vi "VI Test.vi"(6 "Aktion":T1, 8 "error in (no error)":errorcluster caption="Fehler (Eingang, kein Fehler)") -> (0 "error out":errorcluster caption="Fehler (Ausgang)", 1 "Status Test":string, 2 "Fertig":bool, 4 "Aktion":T1, 5 "Test":dbl=30.0, 7 "Warten":dbl)   [LabVIEW 2020, in "EPA 1065.lvlib" / "Interference verificaton 1065-366.lvlib"]
uses:
  Interference verificaton 1065-366.lvlib
  Aktion Test.ctl
  Sprachverwaltung/FGV Aktion Tabelle zerlegen.ctl
  Aktion FGV Interference.ctl
  Aktion Index uebersetzten.ctl
  Seiten/CalGas Aufschaltung/FGV CalGas Aktionen.ctl
  Funktionstasten/Zustaende.ctl
  Funktionstasten/Funktionstasten-Aktion.ctl
  Seiten/CalGas Aufschaltung/Auswahl Aufschaltpunkt.ctl
  PNS/Aktionen FGV Grenzwerte.ctl
  Sprachverwaltung/Sprachverwaltung.lvlib
  Funktionstasten/Funktionstasten.lvlib
  Seiten/CalGas Aufschaltung/CalGas Aufschaltung.lvlib
  PNS/PNS.lvlib
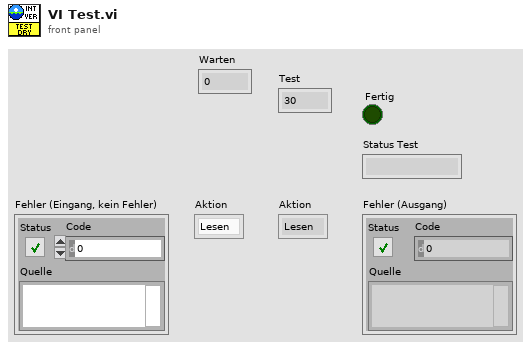
[diagram p1: front panel]
types:
  T1 = typedef "EPA 1065.lvlib/Interference verificaton 1065-366.lvlib/Aktion Test.ctl" = enum16{"Lesen", "ini", "ini - Konz", "Konzentration erreicht", "ini-warten", "ini-Warten-Stabil", "Warten-Stabil", "ini-warten-aufzeichnen", "Warten-Aufzeichnen", "aufzeichnen", "ini-wet", "ini - konz - wet", "Konzentration erreicht - wet", "ini - warten - wet", "warten - wet", "warten - aufzeichnen - wet", "Auswerten", "aufzeichnen - wet"}
  T2 = typedef "CalGas Aufschaltung.lvlib/FGV CalGas Aktionen.ctl" = enum16{"lesen", "Analysator Auswahl", "Def.CalGas", "Aufschaltung CalGas", "laden", "speichern", "KAL extrahieren"}
  T3 = typedef "EPA 1065.lvlib/Interference verificaton 1065-366.lvlib/Aktion Index uebersetzten.ctl" = enum16{"lesen", "schreiben", "auswerten"}
  T4 = typedef "EPA 1065.lvlib/Interference verificaton 1065-366.lvlib/Aktion FGV Interference.ctl" = enum16{"Lesen", "TestKonfig", "TestSetting", "Einheiten", "Ergebnis", "Laden", "Tabelle", "Speichern", "löschen"}
  T5 = typedef "Sprachverwaltung.lvlib/FGV Aktion Tabelle zerlegen.ctl" = enum16{"laden", "vereinzeln", "speichern"}
  T6 = typedef "Funktionstasten.lvlib/Funktionstasten-Aktion.ctl" = enum16{"Initialisieren", "Zustand setzen", "Taste gedrückt", "Fehler speichern", "Lesen", "Manuell", "Remote", "Bitparallel", "Samplepoint", "Zeit Prüfen", "reset Umschalten"}
  T7 = typedef "Funktionstasten.lvlib/Zustaende.ctl" = enum16{"Standby", "Pause", "Eco", "Messen", "Kalibrieren", "Spülen Filter", "Spülen Leitung", "Umgebungsluft", "0-Gas", "Cal-Gas", "CG zu PNS", "-------------", "Init 1", "Init 2", "Init 3", "Init 4", "Messen vorbereiten", "Messen durchführen", "Exit"}
  T8 = typedef "CalGas Aufschaltung.lvlib/Auswahl Aufschaltpunkt.ctl" = enum16{"über Filterblock", "Analysator direkt", "über PNS", "Entnahme", "Gasdivider"}
  T9 = typedef "PNS.lvlib/Aktionen FGV Grenzwerte.ctl" = enum16{"lesen", "Grenzw. schreiben", "Anweisungscode", "IP-Adresse", "laden", "speichern", "Anweisungscode vorgeben"}
  T10 = typedef "CalGas Aufschaltung.lvlib/Aufschaltung CalGas.ctl" = cluster{"Kalibriergas":T11, "Aufschaltpunkt":T8, "Analysator":T12}
  T11 = typedef "Auswahlfeld.ctl" = u16
  T12 = typedef "CalGas Aufschaltung.lvlib/Auswahl Analysator.ctl" = enum16{"FT-IR", "FID", "PMA", "PMA/FID/FT-IR"}
  T13 = typedef "EPA 1065.lvlib/Interference verificaton 1065-366.lvlib/TestKonfig.ctl" = cluster{"CH4:":u16, "Ethane:":u16, "NMHC:":u16, "NMNEHC:":u16, "Komp 1 aktiv:":bool, "Komp 2 aktiv:":bool, "Komp 3 aktiv:":bool, "Komp 4 aktiv:":bool, "Modus":T14, "CG Aufschaltzeit:":dbl, "Interferent 1: CO2":u16, "Interferent 2: H2O":u16, "Interferent 3: CH4":u16, "Interferent 4: C2H6 / C3H8":u16, "Gasflaschen Nr.:":string, "Gasflaschen Nr.: 3":string, "Gasflaschen Nr.: 4":string, "Inter 1 aktiv":bool, "Inter 2 aktiv":bool, "Inter 3 aktiv":bool, "Inter 4 aktiv":bool, "Accuracy":string, "Accuracy 3":string, "Accuracy 4":string, "Konzentration 1:":dbl, "Konzentration 2:":dbl, "Konzentration 3:":dbl, "Konzentration 4:":dbl, "Flow weighted mean 1:":dbl, "Flow weighted mean 2:":dbl, "Flow weighted mean 3:":dbl, "Flow weighted mean 4:":dbl}
  T14 = typedef "EPA 1065.lvlib/Interference verificaton 1065-366.lvlib/Modus.ctl" = u16
  T15 = typedef "String - Ausgabefeld.ctl" = string
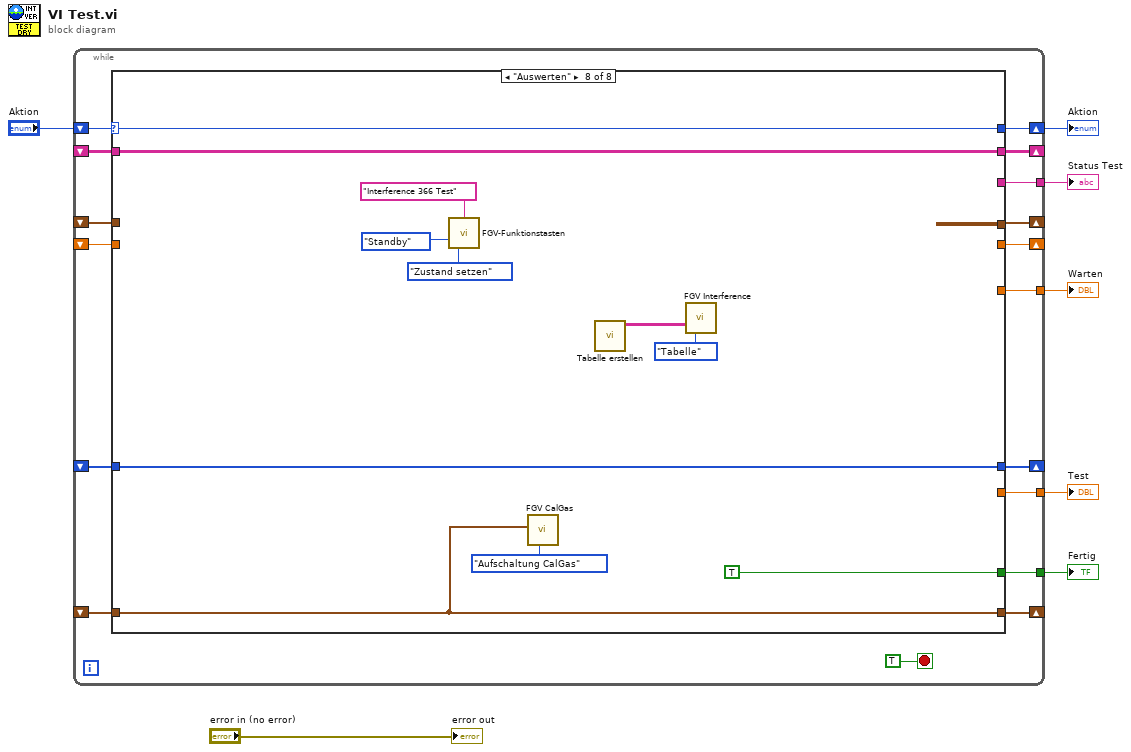
[diagram p0: block diagram]
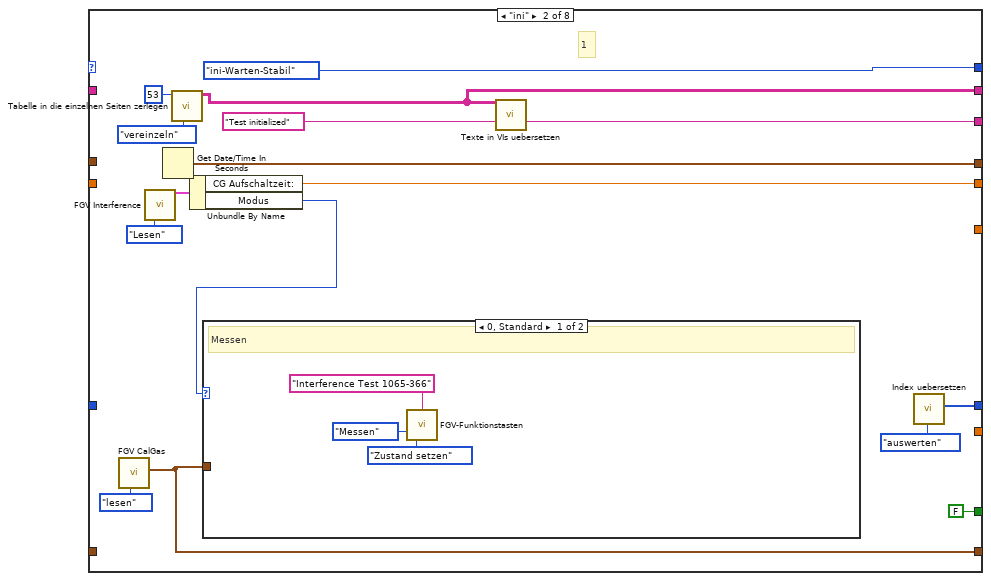
[diagram p3: hidden frame]
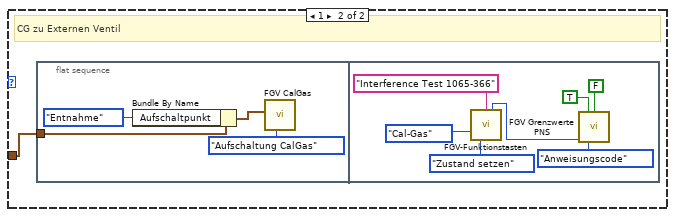
[diagram p4: hidden frame]
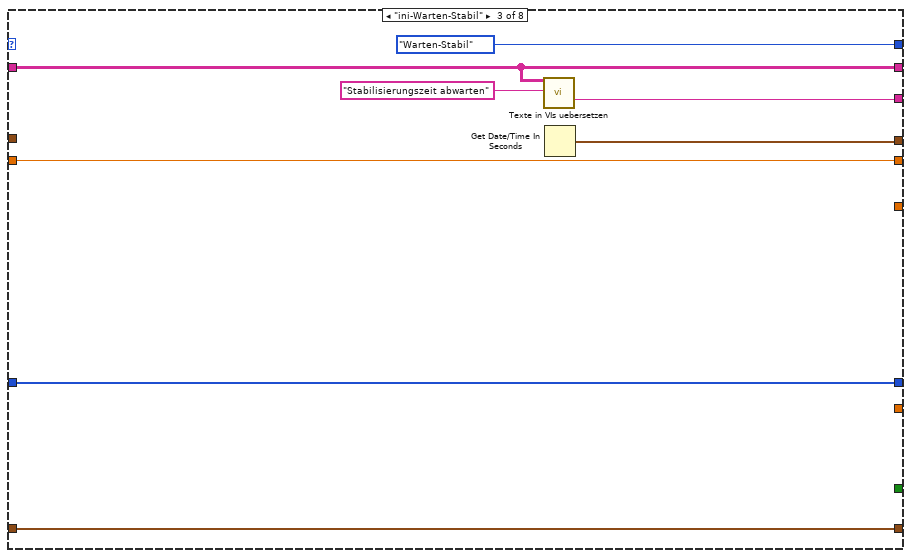
[diagram p5: hidden frame]
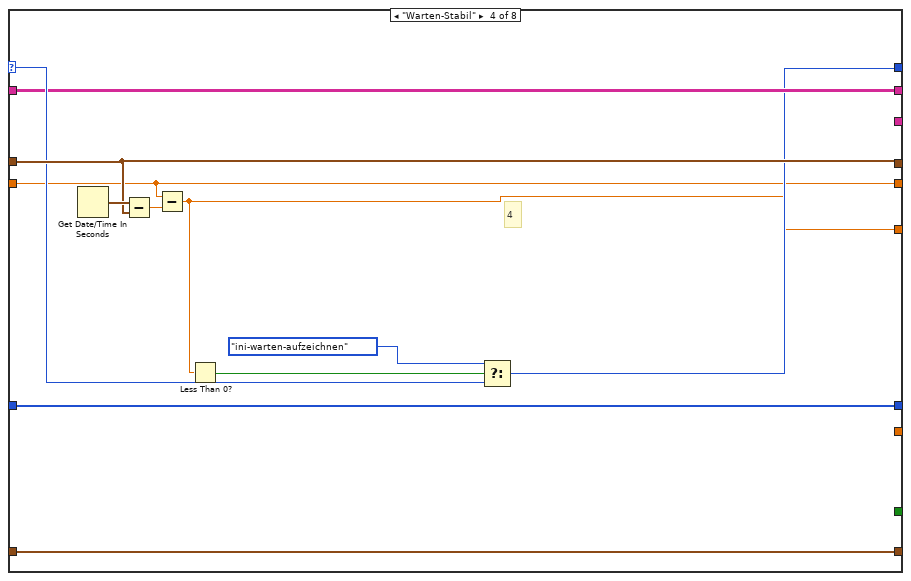
[diagram p6: hidden frame]
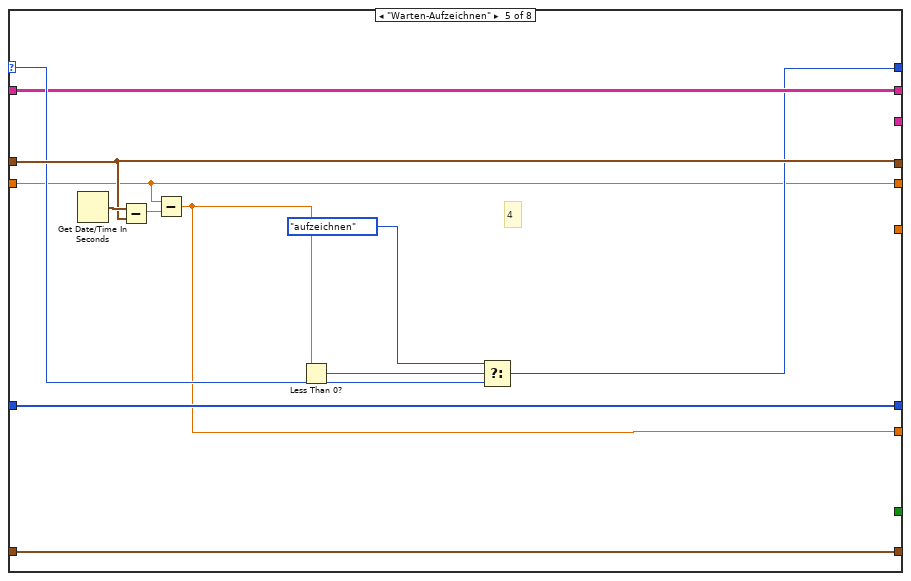
[diagram p7: hidden frame]
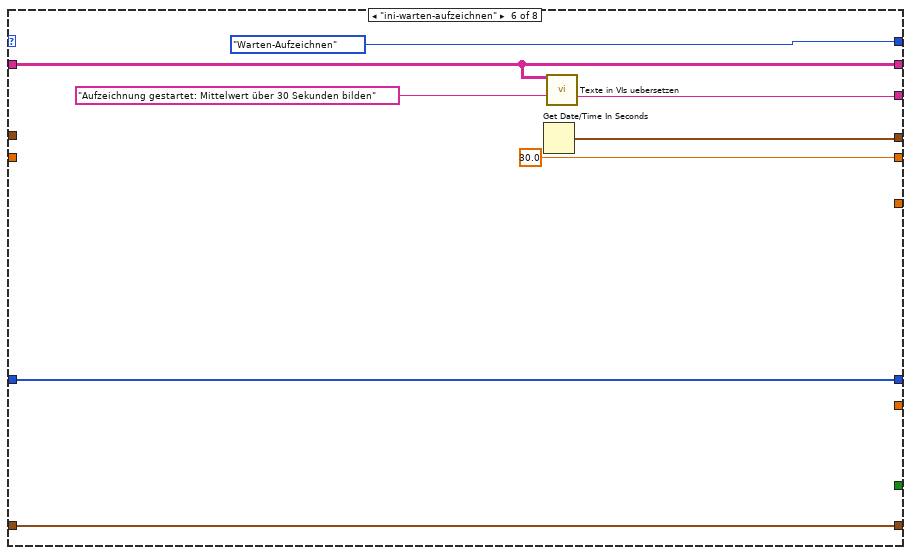
[diagram p8: hidden frame]
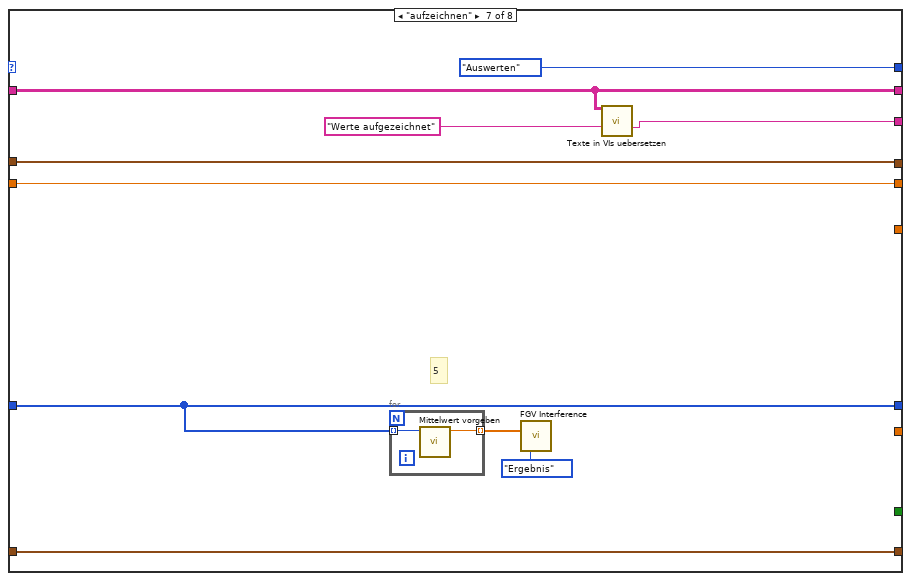
[diagram p9: hidden frame]
diagram:
  n1 = while {
    shift-right: [w23] -> _
    shift-left: _ -> [w22]
    tunnel: [w21] -> w6
    shift-right: [w20] -> _
    shift-left: _ -> [w19]
    shift-right: [w18] -> _
    shift-left: _ -> [w17]
    shift-right: [w16] -> _
    shift-left: _ -> [w15]
    shift-right: [w13] -> w4
    shift-left: "Aktion" -> [w14]
    tunnel: [w12] -> w3
    tunnel: [w11] -> w2
    tunnel: [w10] -> w1
    shift-right: [w9] -> _
    shift-left: _ -> [w8]
    stop <- TRUE stop-if-true
    n2 = case shown="\"Auswerten\"" w14 {
      selector: w14 -> [w26 _ _ w76 w88 _ _ w123]
      tunnel: [w29 w45 w68 w79 w91 w94 w110 _] -> w23
      tunnel: w22 -> [w29 _ _ w79 w91 _ w110 _]
      tunnel: [_ w42 w67 _ _ w100 w103 _] -> w21
      tunnel: [w28 w41 w65 w75 w87 w99 w104 w122] -> w20
      tunnel: w19 -> [w28 _ w65 w75 w87 w99 w104 w122]
      tunnel: [w27 w34 w64 w74 w86 w97 w109 w120] -> w18
      tunnel: w17 -> [w27 _ w64 w74 w86 w97 w109 w120]
      tunnel: [_ w37 w62 w71 w84 30.0 ("CG Aufschaltzeit:") w106 _] -> w16
      tunnel: w15 -> [_ _ w62 w71 w84 _ w106 _]
      tunnel: [w26 Aktion_Test."ini-Warten-Stabil" ("Enum") Aktion_Test."Warten-Stabil" ("Enum") w73 w85 Aktion_Test."Warten-Aufzeichnen" ("Enum") Aktion_Test."Auswerten" ("Enum") w123] -> w13
      tunnel: [_ FALSE ("Erreicht") _ _ _ _ _ TRUE] -> w12
      tunnel: [_ _ _ w70 _ _ _ _] -> w11
      tunnel: [_ _ _ _ w82 _ _ _] -> w10
      tunnel: [w25 w31 w61 w69 w81 w93 w101 w113] -> w9
      tunnel: w8 -> [w25 _ w61 w69 w81 w93 w101 w113]
      frame "Lesen", Default {
      }
      frame "ini" {
        # "1"
        n3 = call "FGV CalGas.vi"("Aktionen"=FGV_CalGas_Aktionen."lesen") -> ("Aufschaltung CalGas"=w31:T10)  [unwired: 6 in, 4 out]
        n4 = call "FGV Interference.vi"("Aktion FGV Interference"=Aktion_FGV_Interference."Lesen") -> ("TestKonfig"=w38:T13)  [unwired: 9 in, 5 out]
        n5 = Get Date/Time In Seconds() -> (seconds since 1Jan1904=w45:timestamp)
        n6 = call "Tabelle in die einzelnen Seiten zerlegen.vi"("Aktion"=FGV_Aktion_Tabelle_zerlegen."vereinzeln", "Index (Seite)"=53) -> ("Sprachliste"=w41:string[][])  [unwired: 7 in, 2 out]
        n7 = Unbundle By Name(w38) -> ("CG Aufschaltzeit:"=w37:dbl, "Modus"=w30:T14)
        n8 = case shown="0, Standard" w30 {
          tunnel: w31 -> [_ w49]
          frame 0, Default {
            # "Messen"
            n9 = call "FGV-Funktionstasten.vi"("Herkunft"="Interference Test 1065-366", "Zustand"=Zustaende."Messen", "Aktion"=Funktionstasten-Aktion."Zustand setzen") -> ()  [unwired: 5 in, 8 out]
          }
          frame 1 {
            # "CG zu Externen Ventil"
            n10 = flat-sequence {
              tunnel: w49 -> [w52]
              frame #0 {
                n11 = Bundle By Name(cluster=w52, "Aufschaltpunkt"=Auswahl_Aufschaltpunkt."Entnahme") -> (w53:T10)
                n12 = call "FGV CalGas.vi"("Aktionen"=FGV_CalGas_Aktionen."Aufschaltung CalGas", "Aufschaltung CalGas"=w53) -> ()  [unwired: 5 in, 5 out]
              }
              frame #1 {
                n13 = call "FGV-Funktionstasten.vi"("Herkunft"="Interference Test 1065-366", "Zustand"=Zustaende."Cal-Gas", "Aktion"=Funktionstasten-Aktion."Zustand setzen") -> ("Samplepoint"=w54:u16)  [unwired: 5 in, 7 out]
                n14 = call "FGV Grenzwerte PNS.vi"("T90"=TRUE ("T90 lüften"), "T90 lüften"=FALSE, "Samplepoint"=w54, "Aktionen FGV Grenzwerte"=Aktionen_FGV_Grenzwerte."Anweisungscode") -> ()  [unwired: 9 in, 3 out]
              }
            }
          }
        }
        n15 = call "Texte in VIs uebersetzen.vi"("Sprachliste"=w41, "String zum Übersetzen"="Test initialized") -> ("String zum Übersetzen"=w42:string)  [unwired: 9 in, 4 out]
        n16 = call "Index uebersetzen.vi"("Aktion"=Aktion_Index_uebersetzten."auswerten") -> ("Komponenten"=w34:i32[])  [unwired: 9 in, 1 out]
      }
      frame "ini-Warten-Stabil" {
        n17 = call "Texte in VIs uebersetzen.vi"("Sprachliste"=w65, "String zum Übersetzen"="Stabilisierungszeit abwarten") -> ("String zum Übersetzen"=w67:string)  [unwired: 9 in, 4 out]
        n18 = Get Date/Time In Seconds() -> (seconds since 1Jan1904=w68:timestamp)
      }
      frame "Warten-Stabil" {
        # "4"
        n19 = Get Date/Time In Seconds() -> (seconds since 1Jan1904=w80:timestamp)
        n20 = Subtract(x=w80, y=w79) -> (x-y=w72:dbl)
        n21 = Subtract(x=w71, y=w72) -> (x-y=w70:dbl)
        n22 = Less Than 0?(x=w70) -> (x < 0?=w77:bool)
        n23 = Select(t=Aktion_Test."ini-warten-aufzeichnen" ("Enum"), s=w77, f=w76) -> (s? t:f=w73:T1)
      }
      frame "Warten-Aufzeichnen" {
        # "4"
        n24 = Get Date/Time In Seconds() -> (seconds since 1Jan1904=w92:timestamp)
        n25 = Subtract(x=w92, y=w91) -> (x-y=w83:dbl)
        n26 = Subtract(x=w84, y=w83) -> (x-y=w82:dbl)
        n27 = Less Than 0?(x=w82) -> (x < 0?=w89:bool)
        n28 = Select(t=Aktion_Test."aufzeichnen" ("Enum"), s=w89, f=w88) -> (s? t:f=w85:T1)
      }
      frame "ini-warten-aufzeichnen" {
        n29 = Get Date/Time In Seconds() -> (seconds since 1Jan1904=w94:timestamp)
        n30 = call "Texte in VIs uebersetzen.vi"("Sprachliste"=w99, "String zum Übersetzen"="Aufzeichnung gestartet: Mittelwert über 30 Sekunden bilden") -> ("String zum Übersetzen"=w100:string)  [unwired: 9 in, 4 out]
      }
      frame "aufzeichnen" {
        # "5"
        n31 = for {
          tunnel: [w112] -> w108 mode=indexing
          tunnel: w109 -> [w111] mode=indexing
          n32 = call "Mittelwert vorgeben.vi"("Komponente"=w111) -> ("Mittelwert"=w112:sgl)  [unwired: 10 in]
        }
        n33 = call "FGV Interference.vi"("Ergebnis"=w108, "Aktion FGV Interference"=Aktion_FGV_Interference."Ergebnis") -> ()  [unwired: 8 in, 6 out]
        n34 = call "Texte in VIs uebersetzen.vi"("Sprachliste"=w104, "String zum Übersetzen"="Werte aufgezeichnet") -> ("String zum Übersetzen"=w103:string)  [unwired: 9 in, 4 out]
      }
      frame "Auswerten" {
        n35 = call "FGV-Funktionstasten.vi"("Herkunft"="Interference 366 Test", "Zustand"=Zustaende."Standby", "Aktion"=Funktionstasten-Aktion."Zustand setzen") -> ()  [unwired: 5 in, 8 out]
        n36 = call "FGV CalGas.vi"("Aktionen"=FGV_CalGas_Aktionen."Aufschaltung CalGas", "Aufschaltung CalGas"=w113) -> ()  [unwired: 5 in, 5 out]
        n37 = call "Tabelle erstellen.vi"() -> ("Tabelle"=w119:T15[][])  [unwired: 11 in]
        n38 = call "FGV Interference.vi"("Tabelle"=w119, "Aktion FGV Interference"=Aktion_FGV_Interference."Tabelle") -> ()  [unwired: 8 in, 6 out]
      }
    }
  }
  "Status Test" <- w6
  "Warten" <- w2
  "Aktion" <- w4
  "Fertig" <- w3
  "Test" <- w1
  "error out" <- "error in (no error)"
